vi "App Top Level Tasks.vi"(8 "error in (no error)":errorcluster, 11 "App in":refnum<class "App.lvclass">) -> (0 "error out":errorcluster, 2 "Top Level Tasks":refnum<class "Task.lvclass">[](array[class]))   [LabVIEW 2020, in "Volatus.lvlib" / "App.lvclass"]
uses:
  App.lvclass
  Task/Task.lvclass
  App.lvclass/App.ctl
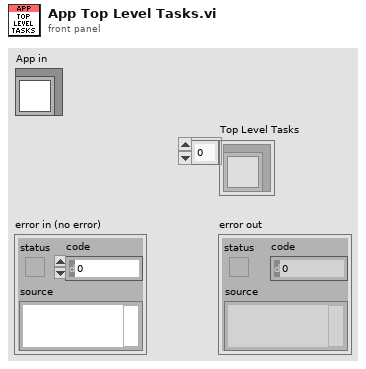
[diagram p1: front panel]
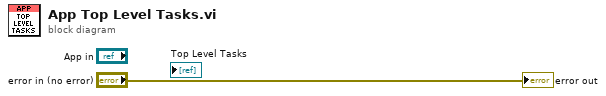
[diagram p0: block diagram]
diagram:
  "error out" <- "error in (no error)"
